vi "Begin Unpolled Mode.vi"(8 "error in (no error)":errorcluster, 11 "Neph in":refnum<class "Nephelometer.lvclass">) -> (0 "error out":errorcluster, 3 "Neph out":refnum<class "Nephelometer.lvclass">)   [LabVIEW 2014, in "Nephelometer.lvclass"]
uses:
  Nephelometer.lvclass
  Nephelometer.lvclass/Nephelometer.ctl
  Accessors/Read Session Handle.vi
  <userlib>/_Session Fwk/Session - Root.lvclass
  Reusable/Session APIs/Text Communication/Text Device Session.lvclass
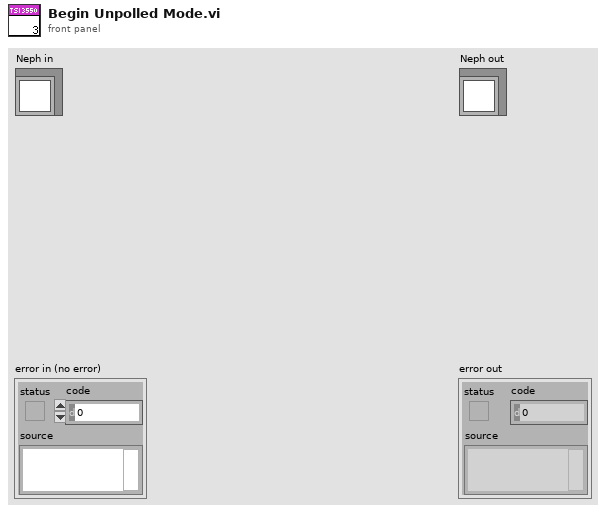
[diagram p1: front panel]
types:
  T1 = typedef "Session - Root.lvclass/Session Handle.ctl" = refnum<data-value>
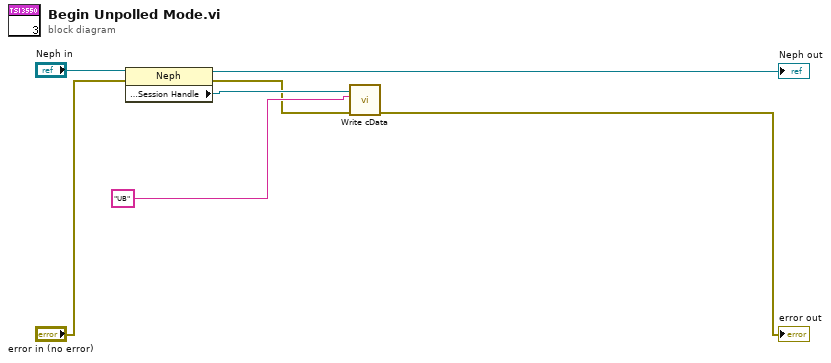
[diagram p0: block diagram]
diagram:
  n1 = property class="Neph"(reference="Neph in", error in="error in (no error)") -> (reference out=→"Neph out":refnum<class "Nephelometer.lvclass">, error out=w2:errorcluster, "Accessors:Session Handle"=w4:T1)
  n2 = call "Write cData.vi"("error in"=w2, "Data"="UB" ("Write - Asynchronous"), "hSession In"=w4) -> ("error out"=→"error out":errorcluster)  [unwired: 7 in, 1 out]
